vi "Update-Create Task DAQmx (SubVI).vi"(0 "Module Configure":T1={"DAQ #"=1, "Module #"=4, "Units"=10065, "input terminal configuration"=-1} {"input terminal configuration" items=["default"=-1, "RSE"=10083, "NRSE"=10078, "Differential"=10106, "Pseudodifferential"=12529]; "Units" items=["Amps"=10342, "From Custom Scale"=10065]}, 3 "Custom Scale Configure":T2={"Pre-Scale MIN"=[0.004, 0.004, 0.004, 0.004, 0.004, 0.004], "Pre-Scale MAX"=[0.02, 0.02, 0.02, 0.02, 0.02, 0.02], "Pre-Scale UNITS"=[10342, 10342, 10342, 10342, 10342, 10342], "Scaled MIN"=[0.0, 0.0, 0.0, 0.0, 0.0, 0.0], "Scaled MAX"=[300.0, 300.0, 300.0, 300.0, 300.0, 300.0], "Scaled UNITS"=["PSI", "PSI", "PSI", "PSI", "PSI", "PSI"]} {"Pre-Scale UNITS" items=["Volts"=10348, "Amps"=10342, "Deg F"=10144, "Deg C"=10143, "Deg R"=10145, "Kelvins"=10325, "Strain"=10299, "Ohms"=10384, "Hz"=10373, "Seconds"=10364, "Meters"=10219, "Inches"=10379, "Degrees"=10146, "Radians"=10273, "g"=10186, "m/s^2"=12470, "Pascals"=10081, "From TEDS"=12516]}, 9 "E-STOP Input":bool) -> (14 "Task OUT":refnum<k21>="cDAQ1Mod4", 16 "Analog Values":dbl[](array[numeric]), 19 "Error OUT":errorcluster)   [LabVIEW 2009]
uses:
  <vilib>/DAQmx/create/channels.llb/DAQmx Create Channel (AI-Current-Basic).vi
  <vilib>/DAQmx/create/scale.llb/DAQmx Create Scale (Map Ranges).vi
  <vilib>/DAQmx/read.llb/DAQmx Read (Analog 1D DBL NChan 1Samp).vi
panel:
  # "Created by Blake Otting\n3/29/2010"
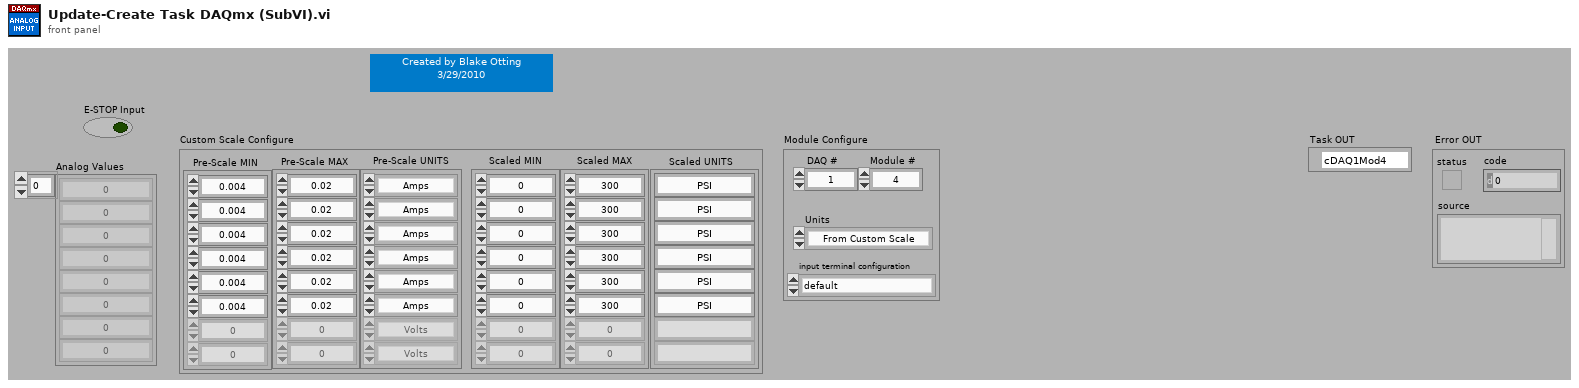
[diagram p1: front panel]
types:
  T1 = cluster{"DAQ #":i32, "Module #":i32, "Units":i32, "input terminal configuration":i32}
  T2 = cluster{"Pre-Scale MIN":dbl[], "Pre-Scale MAX":dbl[], "Pre-Scale UNITS":i32[], "Scaled MIN":dbl[], "Scaled MAX":dbl[], "Scaled UNITS":string[]}
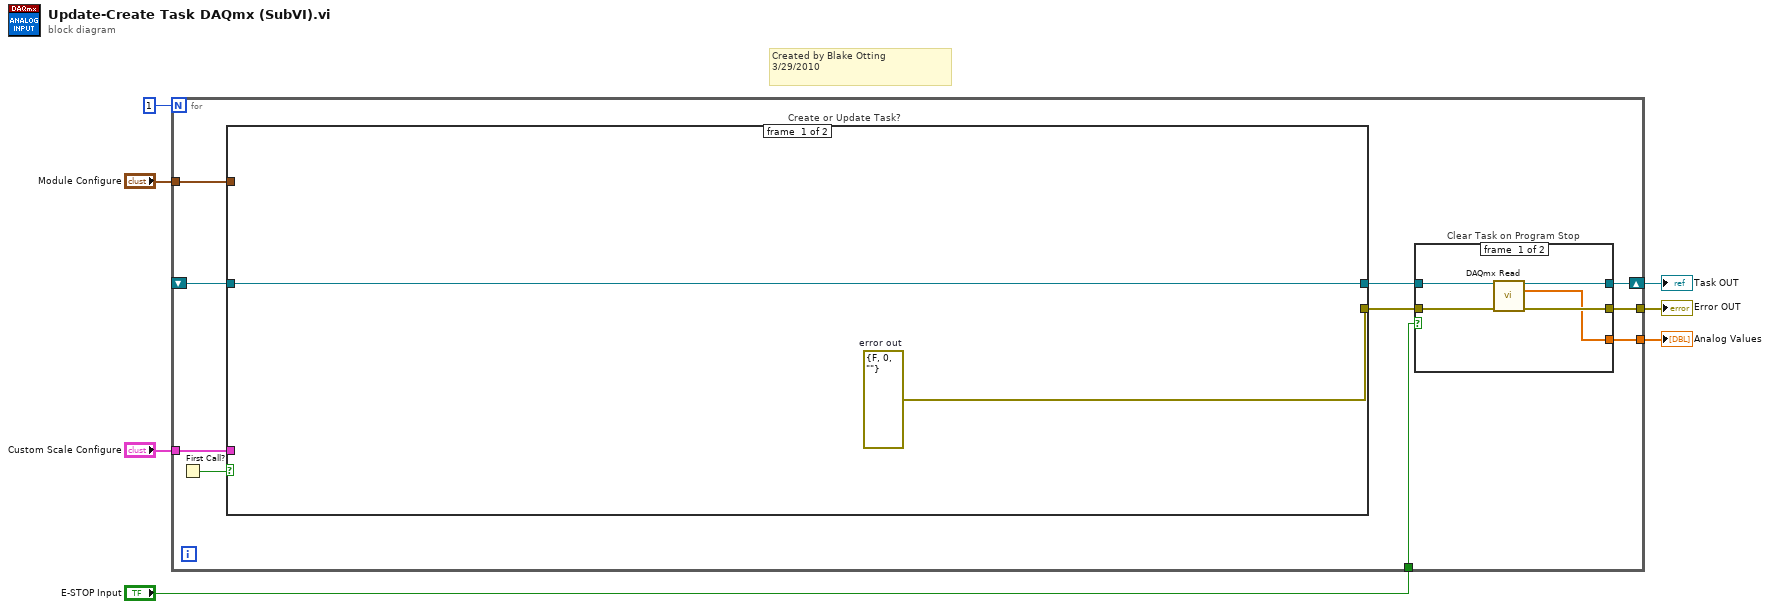
[diagram p0: block diagram]
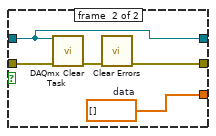
[diagram p2: hidden frame]
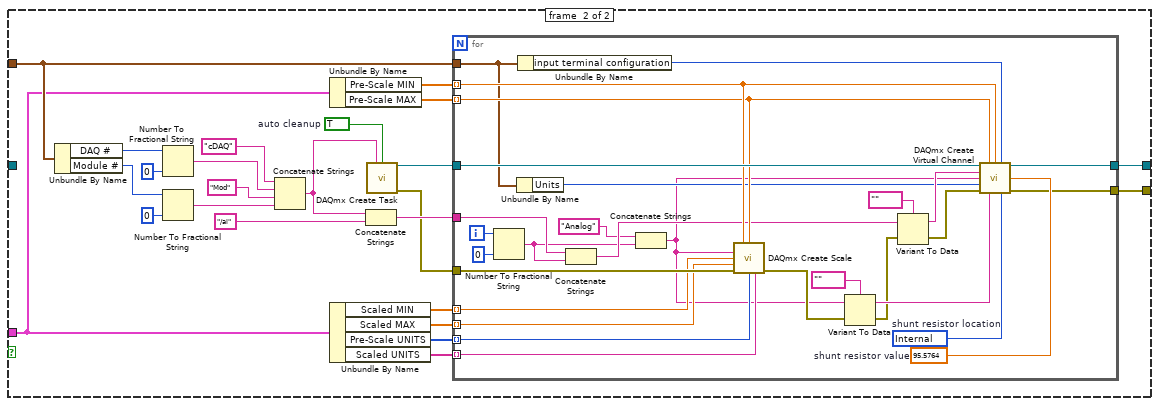
[diagram p3: hidden frame]
diagram:
  # "Created by Blake Otting\n3/29/2010"
  n1 = for {
    N: 1 -> [_]
    tunnel: "Custom Scale Configure" -> [w17]
    tunnel: "Module Configure" -> [w16]
    tunnel: [w9] -> w5
    shift-right: [w10] -> w4
    shift-left: _ -> [w15]
    tunnel: "E-STOP Input" -> [w11]
    tunnel: [w8] -> w1
    n2 = First Call?() -> (First Call?: T/F=w14:bool)
    n3 = case "Create or Update Task?" shown="True" w14 {
      tunnel: [w28 w47] -> w13
      tunnel: [w29 w46] -> w12
      tunnel: w16 -> [_ w42]
      tunnel: w17 -> [_ w37]
      tunnel: w15 -> [w28 _]
      frame #0 {
        w29 = errorcluster {"status"=FALSE, "code"=0, "source"=""}  # error out
      }
      frame #1 {
        w41 = TRUE  # auto cleanup
        n4 = Unbundle By Name(w42) -> ("DAQ #"=w44:i32, "Module #"=w43:i32)
        n5 = Number To Fractional String(number=w44, precision (6)=i16 0) -> (F-format string=w50:string)  [unwired: 2 in]
        n6 = Number To Fractional String(number=w43, precision (6)=i16 0) -> (F-format string=w48:string)  [unwired: 2 in]
        n7 = Concatenate Strings("cDAQ" ("physical channel"), w50, "Mod" ("physical channel"), w48) -> (w38:string)
        n8 = Unbundle By Name(w37) -> ("Pre-Scale MIN"=w30:dbl[], "Pre-Scale MAX"=w45:dbl[])
        n9 = Unbundle By Name(w37) -> ("Scaled MIN"=w36:dbl[], "Scaled MAX"=w35:dbl[], "Pre-Scale UNITS"=w34:i32[], "Scaled UNITS"=w33:string[])
        n10 = Concatenate Strings(w38, "/ai" ("physical channel")) -> (w39:string)
        n11 = call <vilib>:"DAQmx Create Task.vi"("new task name"=w38, "auto cleanup"=w41) -> ("task out"=w32:refnum<k21>, "error out"=w31:errorcluster)  [unwired: 12 in]
        n12 = for {
          tunnel: w30 -> [w68] mode=indexing
          tunnel: w45 -> [w67] mode=indexing
          tunnel: w32 -> [w81]
          tunnel: w31 -> [w66]
          tunnel: w39 -> [w77]
          tunnel: [w72] -> w46
          tunnel: [w71] -> w47
          tunnel: w42 -> [w58]
          tunnel: w36 -> [w63] mode=indexing
          tunnel: w35 -> [w62] mode=indexing
          tunnel: w34 -> [w61] mode=indexing
          tunnel: w33 -> [w60] mode=indexing
          i -> [w79]
          w73 = 95.5764  # shunt resistor value
          w74 = 10200 items=["Internal"=10200, "External"=10167]  # shunt resistor location
          n13 = Number To Fractional String(number=w79, precision (6)=i16 0) -> (F-format string=w56:string)  [unwired: 2 in]
          n14 = Unbundle By Name(w58) -> ("Units"=w57:i32)
          n15 = Unbundle By Name(w58) -> ("input terminal configuration"=w69:i32)
          n16 = Concatenate Strings(w77, w56) -> (w59:string)
          n17 = Concatenate Strings("Analog" ("string"), w56) -> (w54:string)
          n18 = call-poly <vilib>:"DAQmx Create Scale.vi"("pre-scaled minimum"=w68, "pre-scaled maximum"=w67, "name"=w54, "scaled minimum"=w63, "scaled maximum"=w62, "error in"=w66, "pre-scaled units"=w61, "scaled units"=w60) -> ("error out"=w65:errorcluster)  [unwired: 6 in, 1 out]
          n19 = Variant To Data(error in=w65, Variant=w54, type=tag "" ("custom scale name")) -> (error out=w64:errorcluster, data=w75:tag)
          n20 = Variant To Data(error in=w64, Variant=w59, type=tag "" ("physical channels")) -> (error out=w70:errorcluster, data=w82:tag)
          n21 = call-poly <vilib>:"DAQmx Create Virtual Channel.vi"("task in"=w81, "maximum value"=w67, "minimum value"=w68, "input terminal configuration"=w69, "physical channels"=w82, "name to assign"=w54, "external shunt resistor value"=w73, "units"=w57, "error in"=w70, "custom scale name"=w75, "shunt resistor location"=w74) -> ("task out"=w71:refnum<k21>, "error out"=w72:errorcluster)  [unwired: 3 in]
        }
      }
    }
    n22 = case "Clear Task on Program Stop" shown="False" w11 {
      tunnel: w12 -> [w20 w26]
      tunnel: [w19 w25] -> w9
      tunnel: w13 -> [w22 w24]
      tunnel: [w21 w24] -> w10
      tunnel: [w18 w23] -> w8
      frame #0 {
        n23 = call-poly <vilib>:"DAQmx Read.vi"("task/channels in"=w22, "error in"=w20) -> ("task out"=w21:refnum<k21>, "data"=w18:dbl[], "error out"=w19:errorcluster)  [unwired: 11 in]
      }
      frame #1 {
        w23 = dbl[] []  # data
        n24 = call <vilib>:"DAQmx Clear Task.vi"("task in"=w24, "error in"=w26) -> ("error out"=w27:errorcluster)  [unwired: 13 in]
        n25 = call <vilib>:"Clear Errors.vi"("error in (no error)"=w27) -> ("error out"=w25:errorcluster)  [unwired: 6 in]
      }
    }
  }
  "Error OUT" <- w5
  "Task OUT" <- w4
  "Analog Values" <- w1
